vi "SaveRegionDataFile.vi"(2 "Arrays format":string, 3 "Array Titles":string, 4 "Data Type":T1(ring), 5 "no. of arrays":i32, 6 "Actual array lengths":i32, 7 "Region":u32) -> (0 "Path + Filename OUT":string, 1 "Filename OUT":string)   [LabVIEW 2013]
uses:
  global/RunInformation.vi
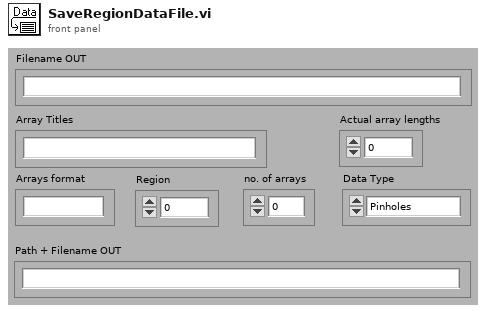
[diagram p1: front panel]
types:
  T1 = enum16{"Pinholes", "Current - voltage", "Voltage - voltage", "CV", "Stability Run", "General", "Interstrip Resistance", "IV Loop", "Combined Tests", "Cis Stability"}
  T2 = enum16{"open", "open or create", "create or replace", "create"}
  T3 = enum32{"Custom", "Standard", "Using Panel", "Using SubVI", "Complete"}
  T4 = cluster{"Manufacturers":string[], "Users":string[], "Device Categories":string[], "MeasurementTypeDirs":string[], "PCNames":string[], "FilePaths":string[], "ThisPCNumber":string, "Full PC Names":string[], "SCTDB Files":string[], "Backuplog directory":string, "Lookup tables":string[], "Projects":string[], "ThisProjectNumber":string, "Institute":string, "java classpath":string, "WWW directories":string[], "BatchFiles":string[], "Logfiles":string[]}
  T5 = cluster{"Measurement No.":u32, "Title":string, "Date & Time":string, "Run Info":string, "Measurement info 1":string, "Measurement info 2":string, "Operator":string, "Device Category":string, "Measurement type":string, "Wafer / Batch No.":string, "Device Description":string, "Serial Number":string, "Probeplan file":string}
  T6 = cluster{"Initial Voltage [V]":dbl, "Final Voltage [V]":dbl, "Number Of Steps":u32, "Step Size [V]":dbl, "Operator":string, "Measurement Description":string, "Step Delay [s]":i32, "Set Current Limit?":bool, "Set Compliance?":bool, "Current Limit [µA]":dbl, "Temperature Readout":enum16{"Read Arduino", "Enter manually"}, "Temperature offset [°C]":dbl, "IV Ramp [V]":dbl, "IV Ramp Delay [s]":i32}
  T7 = cluster{"Initial Voltage [V]":dbl, "Final Voltage [V]":dbl, "Number Of Steps":u32, "Step Size [V]":dbl, "Operator":string, "Measurement Description":string, "Step Delay [s]":i32, "Temperature Readout":enum16{"Read Arduino", "Enter manually"}, "Temperature offset [°C]":dbl, "CV Ramp [V]":dbl, "CV Ramp Delay [s]":i32, "Frequencies [Hz]":i32[], "No. of frequencies":i32, "CV mode":enum16{"Simple CV", "Frequency check", "Full mapping"}, "Set Compliance?":bool, "AC amplitude [V]":dbl, "AC frequency [Hz]":i32, "RC Configuration":u16}
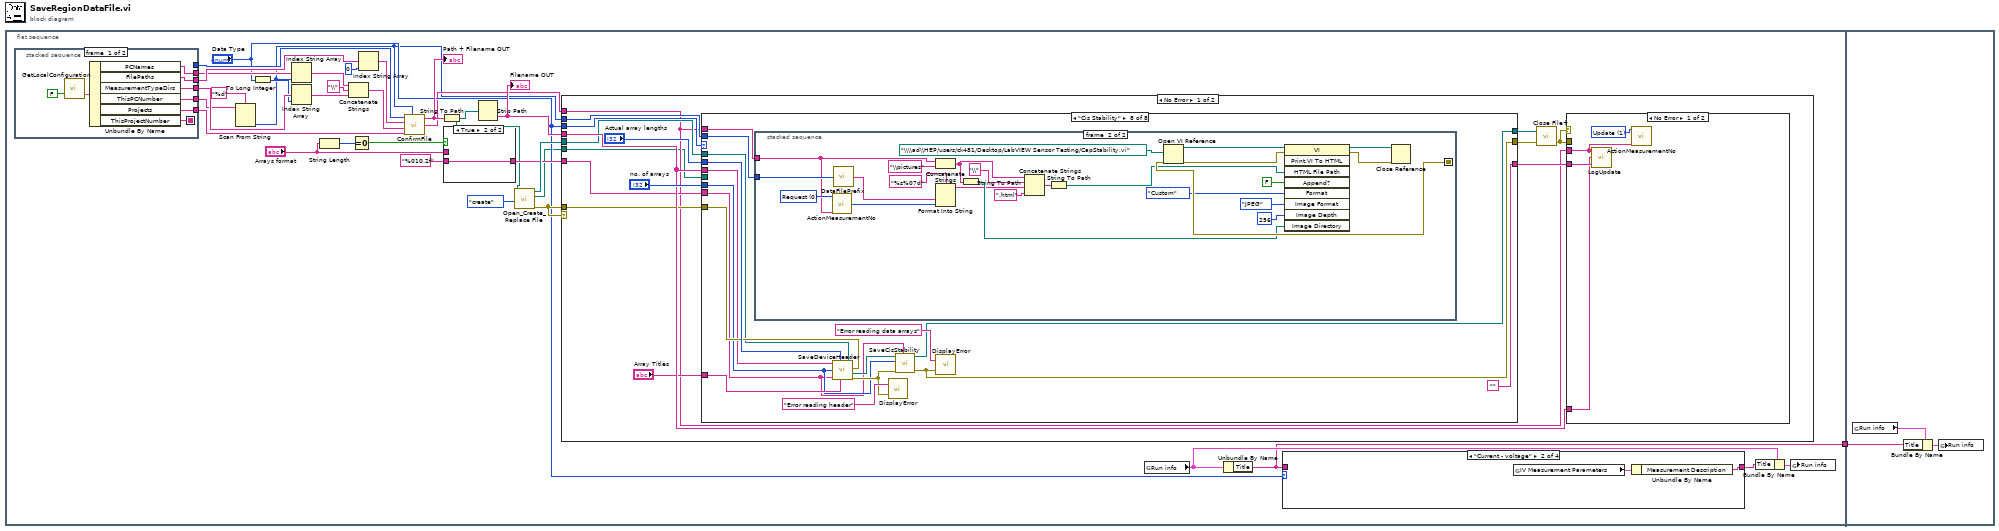
[diagram p0: block diagram]
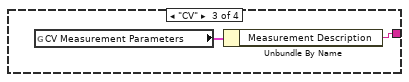
[diagram p3: hidden frame]
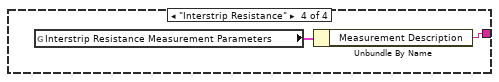
[diagram p4: hidden frame]
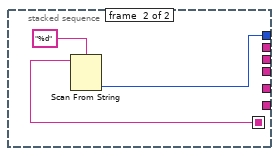
[diagram p5: hidden frame]
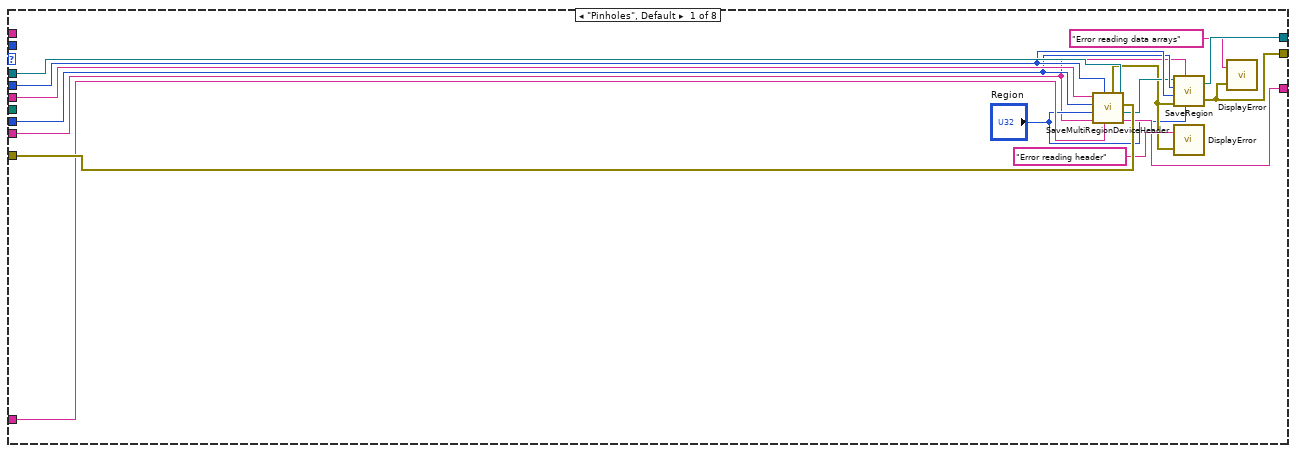
[diagram p7: hidden frame]
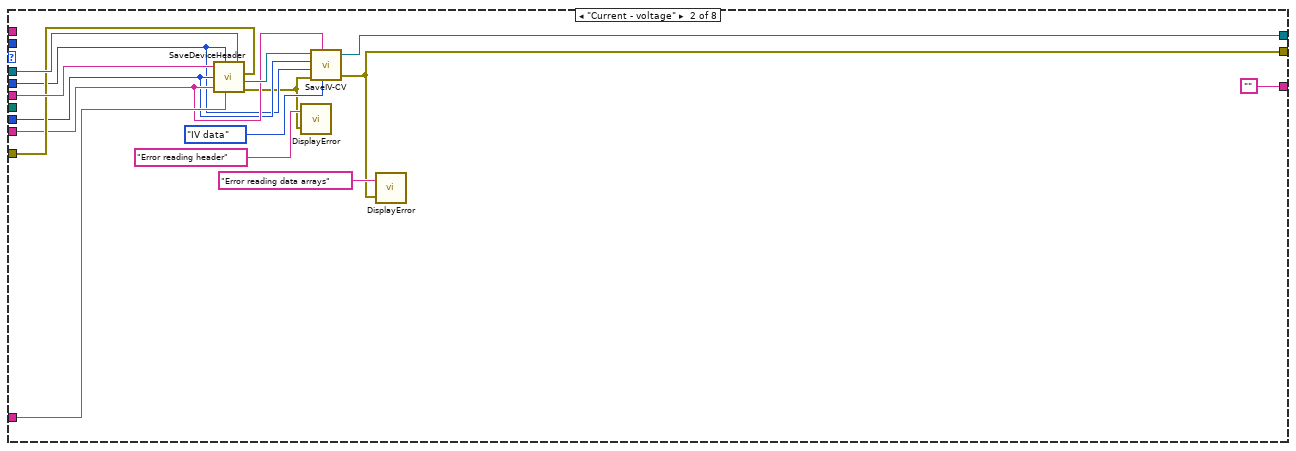
[diagram p8: hidden frame]
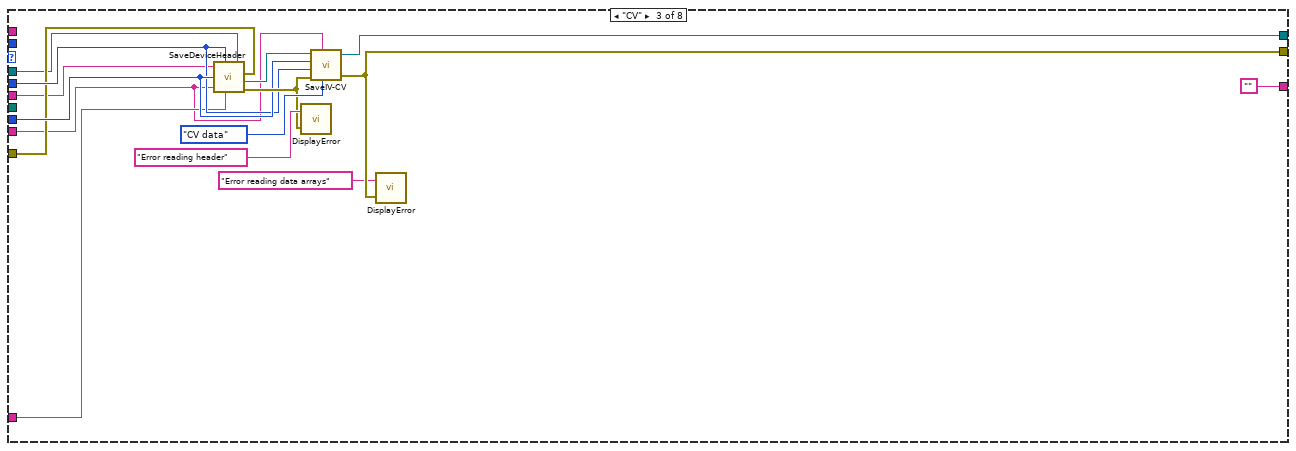
[diagram p9: hidden frame]
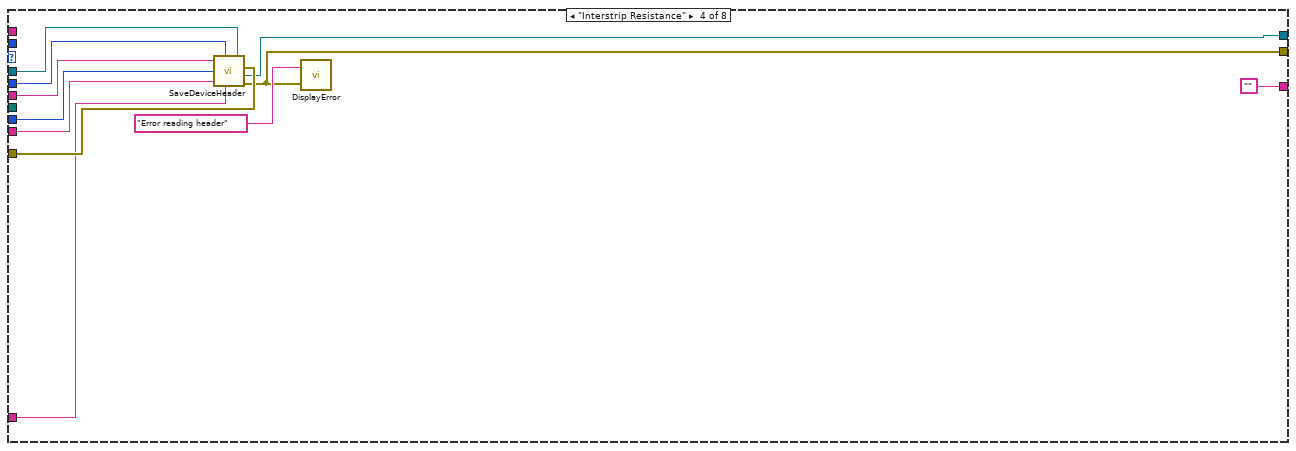
[diagram p10: hidden frame]
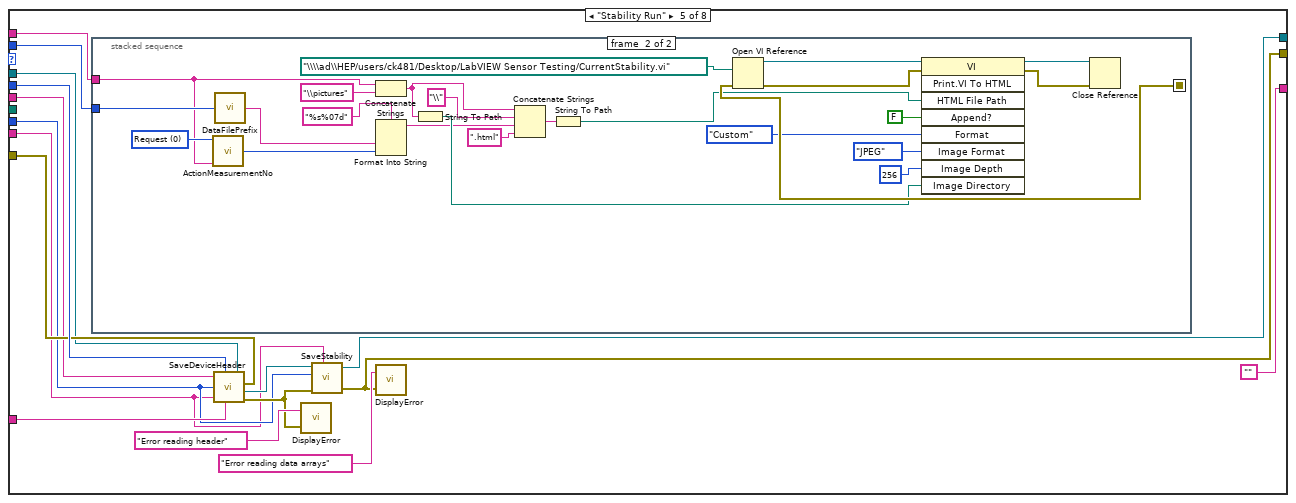
[diagram p11: hidden frame]
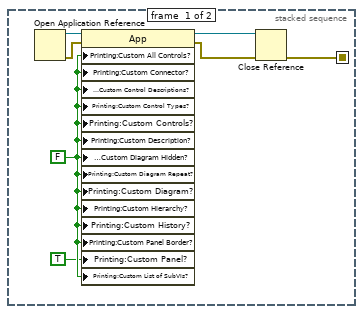
[diagram p12: hidden frame]
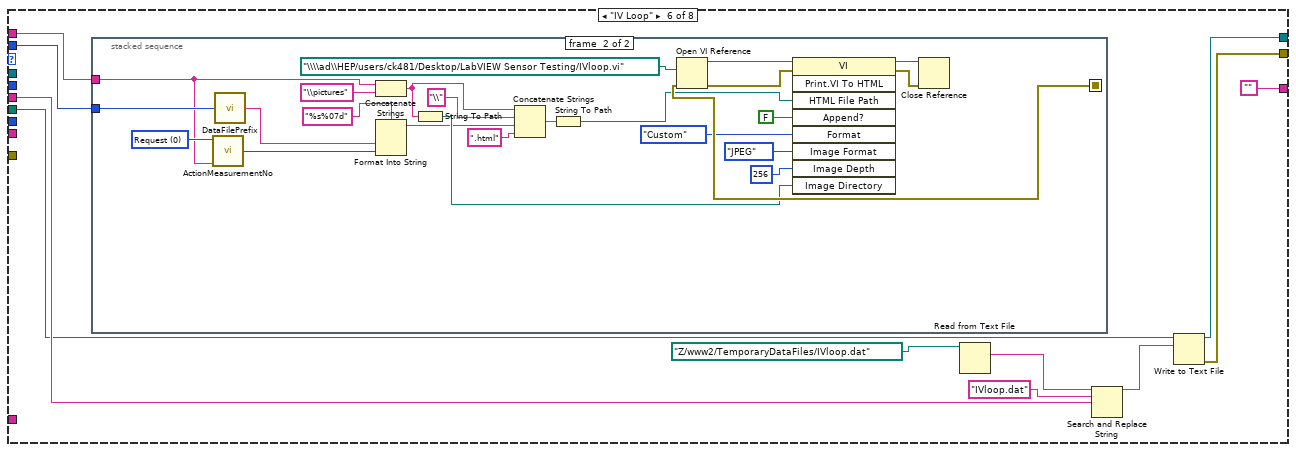
[diagram p13: hidden frame]
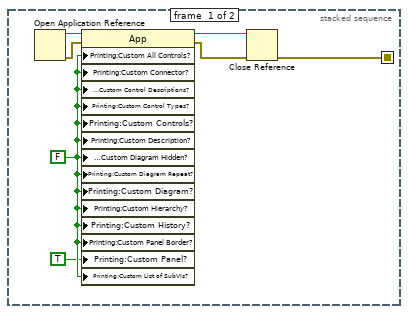
[diagram p14: hidden frame]
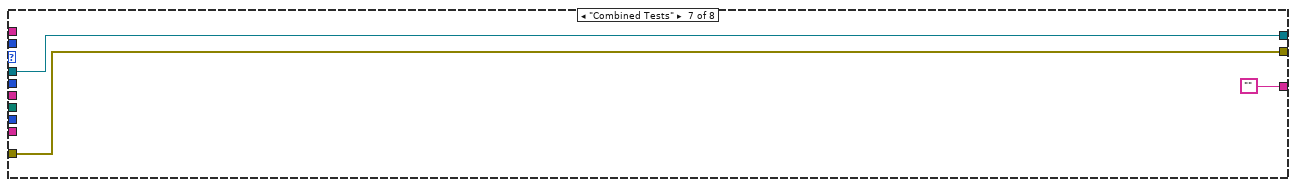
[diagram p15: hidden frame]
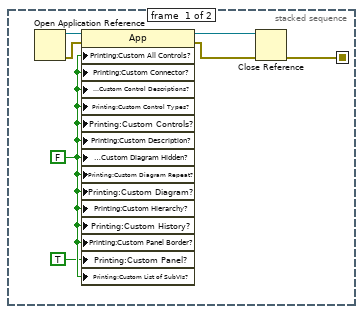
[diagram p16: hidden frame]
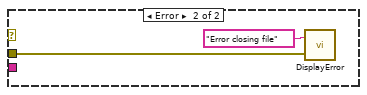
[diagram p17: hidden frame]
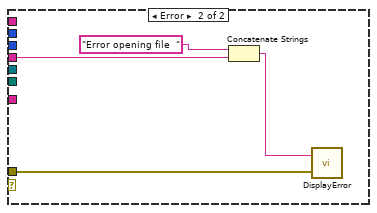
[diagram p18: hidden frame]
diagram:
  n1 = flat-sequence {
    tunnel: [w6] -> w1
    tunnel: w1 -> [w277]
    frame #0 {
      n2 = stacked-sequence {
        seq-local: [w43 _] -> [_ w52]
        tunnel: [w48 _] -> w25
        tunnel: [w47 _] -> w24
        tunnel: [w46 _] -> w23
        tunnel: [w45 _] -> w22
        tunnel: [w44 _] -> w18
        tunnel: [_ w50] -> w15
        frame #0 {
          n3 = call "GetLocalConfiguration.vi"("force read?"=FALSE) -> ("Local Configuration"=w49:T4)  [unwired: 2 in]
          n4 = Unbundle By Name(w49) -> ("PCNames"=w46:string[], "FilePaths"=w48:string[], "MeasurementTypeDirs"=w47:string[], "ThisPCNumber"=w45:string, "Projects"=w44:string[], "ThisProjectNumber"=w43:string)
        }
        frame #1 {
          n5 = Scan From String(format string="%d", input string=w52) -> (output 1=w50:i32)  [unwired: 3 in, 3 out]
        }
      }
      n6 = Scan From String(format string="%d", input string=w22) -> (output 1=w3:i32)  [unwired: 3 in, 3 out]
      n7 = To Long Integer(number="Data Type") -> (32bit integer=w12:i32)
      n8 = Index String Array(1:w3, 2:w23) -> (0:w17:string)  [unwired: 1 in]
      n9 = Index String Array(1:w12, 2:w24) -> (0:w26:string)  [unwired: 1 in]
      n10 = String Length(string="Arrays format") -> (length=w32:i32)
      n11 = Concatenate Strings(w17, "\\", w26) -> (w19:string)
      n12 = Equal To 0?(x=w32) -> (x = 0?=w31:bool)
      n13 = Index String Array(1:0 ("index"), 2:w25) -> (0:w20:string)  [unwired: 1 in]
      n14 = call "ConfirmFile.vi"("Project:"=w15, "f1"=w20, "f2"=w19, "Projects in"=w18, "PCnum"=w3) -> ("Filename:"=w11:string, "Root directory"=w4:string)  [unwired: 1 out]
      "Path + Filename OUT" <- w11
      n15 = String To Path(string=w11) -> (path=w13:path)
      n16 = case shown="True" w31 {
        tunnel: "Arrays format" -> [w53 _]
        tunnel: [w53 w54] -> w29
        tunnel: "%010.2f" -> [_ w54]
        frame False {
        }
        frame True {
        }
      }
      n17 = Strip Path(path=w13) -> (name=w14:string)  [unwired: 1 out]
      "Filename OUT" <- w14
      n18 = call <vilib>:"Open_Create_Replace File.vi"("function (open:0)"=T2."create", "file path"=w13) -> ("error out"=w10:errorcluster, "new file path"=w2:path, "refnum"=w33:refnum<file>)  [unwired: 6 in, 1 out]
      n19 = case shown="No Error" w10 {
        tunnel: w33 -> [w62 _]
        tunnel: w10 -> [w63 w274]
        tunnel: w29 -> [w65 _]
        tunnel: w14 -> [w66 w271]
        tunnel: w4 -> [w56 _]
        tunnel: "Data Type" -> [w69 _]
        tunnel: w3 -> [w57 _]
        tunnel: w2 -> [w55 _]
        frame No Error {
          n20 = case shown="\"Cis Stability\"" w69 {
            tunnel: "no. of arrays" -> [w75 w92 w107 w123 w130 _ _ w222]
            tunnel: "Actual array lengths" -> [w76 w91 w106 w122 w140 _ _ w232]
            tunnel: w66 -> [w83 w99 w101 w118 w129 w177 _ w221]
            tunnel: w65 -> [w70 w93 w100 w117 w128 _ _ w220]
            tunnel: "Array Titles" -> [w82 w96 w102 w119 w141 _ _ w233]
            tunnel: w63 -> [w84 w97 w104 w121 w139 _ w215 w231]
            tunnel: w62 -> [w80 w98 w103 w120 w138 _ w216 w230]
            tunnel: [w79 w94 w112 w115 w133 w174 w216 w225] -> w60
            tunnel: [w78 w86 w109 w116 w132 w173 w215 w224] -> w59
            tunnel: [w74 "" "" "" "" "" "" ""] -> w61
            tunnel: w56 -> [_ _ _ _ w127 w182 _ w219]
            tunnel: w57 -> [_ _ _ _ w126 w181 _ w218]
            tunnel: w55 -> [_ _ _ _ _ w175 _ _]
            frame "Pinholes", Default {
              n21 = call "SaveMultiRegionDeviceHeader.vi"("error in (no error)"=w84, "File Refnum in"=w80, "Array Titles"=w82, "Array Lengths"=w76, "data formats"=w70, "Region"="Region", "no. of arrays"=w75, "Filename"=w83) -> ("Title out"=w74:string, "File Refnum out"=w73:refnum<file>, "error out"=w72:errorcluster)
              n22 = call "SaveRegion.vi"("Region"="Region", "Data formats"=w70, "error in (no error)"=w72, "Number of data points"=w76, "Number of arrays"=w75, "File Refnum in"=w73) -> ("error out"=w78:errorcluster, "File Refnum out"=w79:refnum<file>)
              n23 = call "DisplayError.vi"("Error In"=w72, "Error String In"="Error reading header" ("Error String IN")) -> ()
              n24 = call "DisplayError.vi"("Error In"=w78, "Error String In"="Error reading data arrays" ("Error String IN")) -> ()
            }
            frame "Current - voltage" {
              n25 = call "SaveDeviceHeader.vi"("Filename"=w99, "Array Lengths"=w91, "no. of arrays"=w92, "data formats"=w93, "Array Titles"=w96, "File Refnum in"=w98, "error in (no error)"=w97) -> ("File Refnum out"=w95:refnum<file>, "error out"=w85:errorcluster)
              n26 = call "DisplayError.vi"("Error In"=w85, "Error String In"="Error reading header" ("Error String IN")) -> ()
              n27 = call "SaveIV-CV.vi"("File Refnum in"=w95, "Data formats"=w93, "Number of arrays"=w92, "Number of data points"=w91, "IV/CV data"=enum16{"IV data", "CV data"}."IV data", "error in (no error)"=w85) -> ("File Refnum out"=w94:refnum<file>, "error out"=w86:errorcluster)  [unwired: 1 in]
              n28 = call "DisplayError.vi"("Error In"=w86, "Error String In"="Error reading data arrays" ("Error String IN")) -> ()
            }
            frame "CV" {
              n29 = call "SaveDeviceHeader.vi"("Filename"=w101, "Array Lengths"=w106, "no. of arrays"=w107, "data formats"=w100, "Array Titles"=w102, "File Refnum in"=w103, "error in (no error)"=w104) -> ("File Refnum out"=w105:refnum<file>, "error out"=w110:errorcluster)
              n30 = call "DisplayError.vi"("Error In"=w110, "Error String In"="Error reading header" ("Error String IN")) -> ()
              n31 = call "SaveIV-CV.vi"("File Refnum in"=w105, "Data formats"=w100, "Number of arrays"=w107, "Number of data points"=w106, "IV/CV data"=enum16{"IV data", "CV data"}."CV data", "error in (no error)"=w110) -> ("File Refnum out"=w112:refnum<file>, "error out"=w109:errorcluster)  [unwired: 1 in]
              n32 = call "DisplayError.vi"("Error In"=w109, "Error String In"="Error reading data arrays" ("Error String IN")) -> ()
            }
            frame "Interstrip Resistance" {
              n33 = call "SaveDeviceHeader.vi"("Filename"=w118, "Array Lengths"=w122, "no. of arrays"=w123, "data formats"=w117, "Array Titles"=w119, "File Refnum in"=w120, "error in (no error)"=w121) -> ("File Refnum out"=w115:refnum<file>, "error out"=w116:errorcluster)
              n34 = call "DisplayError.vi"("Error In"=w116, "Error String In"="Error reading header" ("Error String IN")) -> ()
            }
            frame "Stability Run" {
              n35 = stacked-sequence {
                seq-local: [w142 _] -> [_ w171]
                tunnel: w127 -> [_ w151]
                tunnel: w126 -> [_ w156]
                frame #0 {
                  w148 = FALSE ("Pr.CustAllCtls?")
                  n36 = Open Application Reference() -> (0:w145:errorcluster, 3:w146:refnum<vi>)  [unwired: 4 in]
                  n37 = property class="App"(reference=w146, error in=w145, "Printing:Custom All Controls?"=w148, "Printing:Custom Connector?"=w148, "Printing:Custom Control Descriptions?"=w148, "Printing:Custom Control Types?"=w148, "Printing:Custom Controls?"=w148, "Printing:Custom Description?"=w148, "Printing:Custom Diagram Hidden?"=w148, "Printing:Custom Diagram Repeat?"=w148, "Printing:Custom Diagram?"=w148, "Printing:Custom Hierarchy?"=w148, "Printing:Custom History?"=w148, "Printing:Custom Panel Border?"=w148, "Printing:Custom Panel?"=TRUE ("Pr.CustPanel?"), "Printing:Custom List of SubVIs?"=w148) -> (reference out=w144:refnum<vi>, error out=w143:errorcluster)
                  n38 = Close Reference(reference=w144, error in (no error)=w143) -> (error out=w142:errorcluster)
                }
                frame #1 {
                  w158 = u16 0 items=["Request", "Update"] ("Mode:")
                  n39 = call "ActionMeasurementNo.vi"("Root Directory IN"=w151, "Mode:"=w158) -> ("Next Measurement Number"=w160:i32)  [unwired: 2 in]
                  n40 = call "DataFilePrefix.vi"("PC number IN"=w156) -> ("File prefix OUT"=w159:string)
                  n41 = Concatenate Strings(w151, "\\pictures" ("Substring")) -> (w149:string)
                  n42 = Format Into String(format string="%s%07d", w159, w160) -> (resulting string=w155:string)  [unwired: 2 in, 1 out]
                  n43 = String To Path(string=w149) -> (path=w162:path)
                  n44 = Concatenate Strings(w149, "\\" ("Substring"), w155, ".html") -> (w170:string)
                  n45 = String To Path(string=w170) -> (path=w169:path)
                  n46 = Open VI Reference(vi path=path "\\\\ad\\HEP/users/ck481/Desktop/LabVIEW Sensor Testing/CurrentStability.vi", error in (no error)=w171) -> (vi reference=w168:refnum<vi>, error out=w167:errorcluster)  [unwired: 4 in]
                  n47 = invoke class="VI" method="Print.VI To HTML"(reference=w168, error in=w167, "HTML File Path"=w169, "Append?"=FALSE, "Format"=T3."Custom", "Image Format"=enum32{"PNG", "JPEG", "GIF"}."JPEG", "Image Depth"=256, "Image Directory"=w162) -> (reference out=w161:refnum<vi>, error out=w153:errorcluster)  [unwired: 1 in, 7 out]
                  n48 = Close Reference(reference=w161, error in (no error)=w153) -> ()  [unwired: 1 out]
                }
              }
              n49 = call "SaveDeviceHeader.vi"("Filename"=w129, "Array Lengths"=w140, "no. of arrays"=w130, "data formats"=w128, "Array Titles"=w141, "File Refnum in"=w138, "error in (no error)"=w139) -> ("File Refnum out"=w136:refnum<file>, "error out"=w135:errorcluster)
              n50 = call "DisplayError.vi"("Error In"=w135, "Error String In"="Error reading header" ("Error String IN")) -> ()
              n51 = call "SaveStability.vi"("File Refnum in"=w136, "Data formats"=w128, "Number of arrays"=w130, "error in (no error)"=w135) -> ("File Refnum out"=w133:refnum<file>, "error out"=w132:errorcluster)  [unwired: 3 in]
              n52 = call "DisplayError.vi"("Error In"=w132, "Error String In"="Error reading data arrays" ("Error String IN")) -> ()
            }
            frame "IV Loop" {
              n53 = stacked-sequence {
                seq-local: [w184 _] -> [_ w213]
                tunnel: w182 -> [_ w193]
                tunnel: w181 -> [_ w198]
                frame #0 {
                  w190 = FALSE ("Pr.CustAllCtls?")
                  n54 = Open Application Reference() -> (0:w187:errorcluster, 3:w188:refnum<vi>)  [unwired: 4 in]
                  n55 = property class="App"(reference=w188, error in=w187, "Printing:Custom All Controls?"=w190, "Printing:Custom Connector?"=w190, "Printing:Custom Control Descriptions?"=w190, "Printing:Custom Control Types?"=w190, "Printing:Custom Controls?"=w190, "Printing:Custom Description?"=w190, "Printing:Custom Diagram Hidden?"=w190, "Printing:Custom Diagram Repeat?"=w190, "Printing:Custom Diagram?"=w190, "Printing:Custom Hierarchy?"=w190, "Printing:Custom History?"=w190, "Printing:Custom Panel Border?"=w190, "Printing:Custom Panel?"=TRUE ("Pr.CustPanel?"), "Printing:Custom List of SubVIs?"=w190) -> (reference out=w186:refnum<vi>, error out=w185:errorcluster)
                  n56 = Close Reference(reference=w186, error in (no error)=w185) -> (error out=w184:errorcluster)
                }
                frame #1 {
                  w200 = u16 0 items=["Request", "Update"] ("Mode:")
                  n57 = call "ActionMeasurementNo.vi"("Root Directory IN"=w193, "Mode:"=w200) -> ("Next Measurement Number"=w202:i32)  [unwired: 2 in]
                  n58 = call "DataFilePrefix.vi"("PC number IN"=w198) -> ("File prefix OUT"=w201:string)
                  n59 = Concatenate Strings(w193, "\\pictures" ("Substring")) -> (w191:string)
                  n60 = Format Into String(format string="%s%07d", w201, w202) -> (resulting string=w197:string)  [unwired: 2 in, 1 out]
                  n61 = String To Path(string=w191) -> (path=w204:path)
                  n62 = Concatenate Strings(w191, "\\" ("Substring"), w197, ".html") -> (w212:string)
                  n63 = String To Path(string=w212) -> (path=w211:path)
                  n64 = Open VI Reference(vi path=path "\\\\ad\\HEP/users/ck481/Desktop/LabVIEW Sensor Testing/IVloop.vi", error in (no error)=w213) -> (vi reference=w210:refnum<vi>, error out=w209:errorcluster)  [unwired: 4 in]
                  n65 = invoke class="VI" method="Print.VI To HTML"(reference=w210, error in=w209, "HTML File Path"=w211, "Append?"=FALSE, "Format"=T3."Custom", "Image Format"=enum32{"PNG", "JPEG", "GIF"}."JPEG", "Image Depth"=256, "Image Directory"=w204) -> (reference out=w203:refnum<vi>, error out=w195:errorcluster)  [unwired: 1 in, 7 out]
                  n66 = Close Reference(reference=w203, error in (no error)=w195) -> ()  [unwired: 1 out]
                }
              }
              n67 = Read from Text File(file (use dialog)=path "Z:/www2/TemporaryDataFiles/IVloop.dat") -> (text=w179:string)  [unwired: 3 in, 3 out]
              n68 = Search and Replace String(input string=w179, search string="IVloop.dat", replace string=w177) -> (result string=w176:string)  [unwired: 5 in, 3 out]
              n69 = Write to Text File(file (use dialog)=w175, text=w176) -> (refnum out=w174:refnum<file>, error out=w173:errorcluster)  [unwired: 2 in, 1 out]
            }
            frame "Combined Tests" {
            }
            frame "Cis Stability" {
              n70 = stacked-sequence {
                seq-local: [w234 _] -> [_ w263]
                tunnel: w219 -> [_ w243]
                tunnel: w218 -> [_ w248]
                frame #0 {
                  w240 = FALSE ("Pr.CustAllCtls?")
                  n71 = Open Application Reference() -> (0:w237:errorcluster, 3:w238:refnum<vi>)  [unwired: 4 in]
                  n72 = property class="App"(reference=w238, error in=w237, "Printing:Custom All Controls?"=w240, "Printing:Custom Connector?"=w240, "Printing:Custom Control Descriptions?"=w240, "Printing:Custom Control Types?"=w240, "Printing:Custom Controls?"=w240, "Printing:Custom Description?"=w240, "Printing:Custom Diagram Hidden?"=w240, "Printing:Custom Diagram Repeat?"=w240, "Printing:Custom Diagram?"=w240, "Printing:Custom Hierarchy?"=w240, "Printing:Custom History?"=w240, "Printing:Custom Panel Border?"=w240, "Printing:Custom Panel?"=TRUE ("Pr.CustPanel?"), "Printing:Custom List of SubVIs?"=w240) -> (reference out=w236:refnum<vi>, error out=w235:errorcluster)
                  n73 = Close Reference(reference=w236, error in (no error)=w235) -> (error out=w234:errorcluster)
                }
                frame #1 {
                  w250 = u16 0 items=["Request", "Update"] ("Mode:")
                  n74 = call "ActionMeasurementNo.vi"("Root Directory IN"=w243, "Mode:"=w250) -> ("Next Measurement Number"=w252:i32)  [unwired: 2 in]
                  n75 = call "DataFilePrefix.vi"("PC number IN"=w248) -> ("File prefix OUT"=w251:string)
                  n76 = Concatenate Strings(w243, "\\pictures" ("Substring")) -> (w241:string)
                  n77 = Format Into String(format string="%s%07d", w251, w252) -> (resulting string=w247:string)  [unwired: 2 in, 1 out]
                  n78 = String To Path(string=w241) -> (path=w254:path)
                  n79 = Concatenate Strings(w241, "\\" ("Substring"), w247, ".html") -> (w262:string)
                  n80 = String To Path(string=w262) -> (path=w261:path)
                  n81 = Open VI Reference(vi path=path "\\\\ad\\HEP/users/ck481/Desktop/LabVIEW Sensor Testing/CapStability.vi", error in (no error)=w263) -> (vi reference=w260:refnum<vi>, error out=w259:errorcluster)  [unwired: 4 in]
                  n82 = invoke class="VI" method="Print.VI To HTML"(reference=w260, error in=w259, "HTML File Path"=w261, "Append?"=FALSE, "Format"=T3."Custom", "Image Format"=enum32{"PNG", "JPEG", "GIF"}."JPEG", "Image Depth"=256, "Image Directory"=w254) -> (reference out=w253:refnum<vi>, error out=w245:errorcluster)  [unwired: 1 in, 7 out]
                  n83 = Close Reference(reference=w253, error in (no error)=w245) -> ()  [unwired: 1 out]
                }
              }
              n84 = call "SaveDeviceHeader.vi"("Filename"=w221, "Array Lengths"=w232, "no. of arrays"=w222, "data formats"=w220, "Array Titles"=w233, "File Refnum in"=w230, "error in (no error)"=w231) -> ("File Refnum out"=w228:refnum<file>, "error out"=w227:errorcluster)
              n85 = call "DisplayError.vi"("Error In"=w227, "Error String In"="Error reading header" ("Error String IN")) -> ()
              n86 = call "SaveCisStability.vi"("File Refnum in"=w228, "Data formats"=w220, "Number of arrays"=w222, "error in (no error)"=w227) -> ("File Refnum out"=w225:refnum<file>, "error out"=w224:errorcluster)  [unwired: 3 in]
              n87 = call "DisplayError.vi"("Error In"=w224, "Error String In"="Error reading data arrays" ("Error String IN")) -> ()
            }
          }
          n88 = call <vilib>:"Close File+.vi"("error in (no error)"=w59, "refnum"=w60) -> ("error out"=w58:errorcluster)  [unwired: 3 in, 2 out]
          n89 = case shown="No Error" w58 {
            tunnel: w58 -> [_ w270]
            tunnel: w56 -> [w265 _]
            tunnel: w66 -> [w266 _]
            tunnel: w61 -> [w267 _]
            frame No Error {
              w268 = u16 1 items=["Request", "Update"] ("Mode:")
              n90 = call "LogUpdate.vi"("Optional title"=w267, "Short filename"=w266, "Root Directory IN"=w265) -> ()
              n91 = call "ActionMeasurementNo.vi"("Root Directory IN"=w265, "Mode:"=w268) -> ()  [unwired: 2 in, 1 out]
            }
            frame Error {
              n92 = call "DisplayError.vi"("Error In"=w270, "Error String In"="Error closing file" ("Error String IN")) -> ()
            }
          }
        }
        frame Error {
          n93 = Concatenate Strings("Error opening file  " ("Error String IN"), w271) -> (w272:string)
          n94 = call "DisplayError.vi"("Error In"=w274, "Error String In"=w272) -> ()
        }
      }
      n95 = global read "RunInformation.vi" "Run info"() -> (w8:T5)
      n96 = Unbundle By Name(w8) -> ("Title"=w6:string)
      n97 = case shown="\"Current - voltage\"" "Data Type" {
        tunnel: [w35 w36 w38 w40] -> w7
        tunnel: w6 -> [w35 _ _ _]
        frame "Pinholes", Default {
        }
        frame "Current - voltage" {
          n98 = global read "RunInformation.vi" "IV Measurement Parameters"() -> (w37:T6)
          n99 = Unbundle By Name(w37) -> ("Measurement Description"=w36:string)
        }
        frame "CV" {
          n100 = global read "RunInformation.vi" "CV Measurement Parameters"() -> (w39:T7)
          n101 = Unbundle By Name(w39) -> ("Measurement Description"=w38:string)
        }
        frame "Interstrip Resistance" {
          n102 = global read "RunInformation.vi" "Interstrip Resistance Measurement Parameters"() -> (w41:T6)
          n103 = Unbundle By Name(w41) -> ("Measurement Description"=w40:string)
        }
      }
      n104 = Bundle By Name(cluster=w8, "Title"=w7) -> (w5:T5)
      n105 = global write "RunInformation.vi" "Run info"(w5) -> ()
    }
    frame #1 {
      n106 = global read "RunInformation.vi" "Run info"() -> (w275:T5)
      n107 = Bundle By Name(cluster=w275, "Title"=w277) -> (w276:T5)
      n108 = global write "RunInformation.vi" "Run info"(w276) -> ()
    }
  }
